vi "Circular Count (SubVI).vi"(7 "Max. Count":u16, 11 "Count In":u16) -> (3 "Count Out":u16)   [LabVIEW 2015]
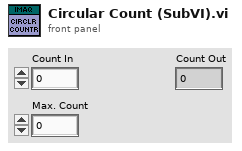
[diagram p1: front panel]
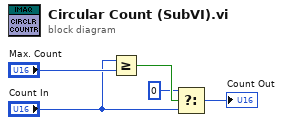
[diagram p0: block diagram]
diagram:
  n1 = Greater Or Equal?(x="Count In", y="Max. Count") -> (x >= y?=w4:bool)
  n2 = Select(t=u16 0, s=w4, f="Count In") -> (s? t:f=→"Count Out":u16)
